vi "SMUVoltage.vi"() -> ()   [LabVIEW 2020]
uses:
  <instrlib>/niDCPower/nidcpower.llb/niDCPower Output Function.ctl
  <instrlib>/niDCPower/nidcpower.llb/niDCPower Measurement Type.ctl
panel:
  out "measurement":dbl format="%_6g"
  in  "instrument handle":refnum<k15>="NI_SMU1"
  in  "error in (no error)":errorcluster
  out "error out":errorcluster
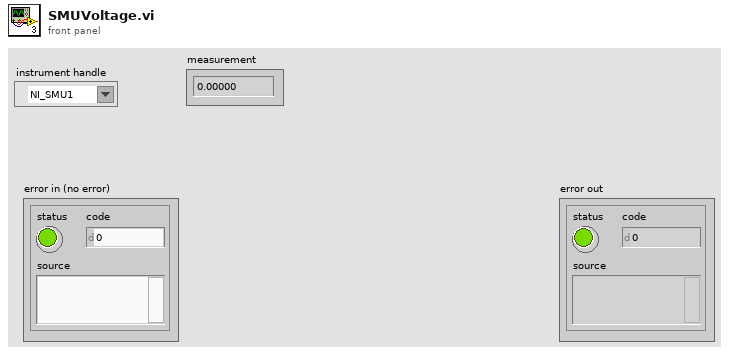
[diagram p1: front panel]
types:
  T1 = typedef "niDCPower Measurement Type.ctl" = i32
  T2 = typedef "niDCPower Output Function.ctl" = i32
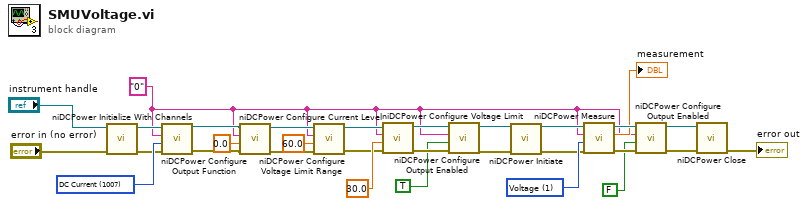
[diagram p0: block diagram]
diagram:
  w18 = T1 1 items=["Current", "Voltage"] ("measurement type")
  w2 = "0" ("channel name")
  w26 = T2 1007 items=["DC Voltage"=1006, "DC Current"=1007, "Pulse Voltage"=1049, "Pulse Current"=1050] ("output function")
  n1 = call <instrlib>:"niDCPower Initialize With Channels.vi"("error in (no error)"="error in (no error)", "resource name"="instrument handle") -> ("error out"=w25:errorcluster, "instrument handle out"=w27:refnum<k15>)  [unwired: 8 in]
  n2 = call <instrlib>:"niDCPower Configure Output Function.vi"("error in (no error)"=w25, "output function"=w26, "channel name"=w2, "instrument handle"=w27) -> ("error out"=w23:errorcluster, "instrument handle out"=w24:refnum<k15>)  [unwired: 6 in]
  n3 = call <instrlib>:"niDCPower Configure Current Level.vi"("error in (no error)"=w23, "current level"=0.0, "channel name"=w2, "instrument handle"=w24) -> ("error out"=w6:errorcluster, "instrument handle out"=w5:refnum<k15>)  [unwired: 6 in]
  n4 = call <instrlib>:"niDCPower Configure Voltage Limit Range.vi"("error in (no error)"=w6, "voltage limit range"=60.0, "channel name"=w2, "instrument handle"=w5) -> ("error out"=w3:errorcluster, "instrument handle out"=w4:refnum<k15>)  [unwired: 6 in]
  n5 = call <instrlib>:"niDCPower Configure Voltage Limit.vi"("error in (no error)"=w3, "voltage limit"=30.0, "channel name"=w2, "instrument handle"=w4) -> ("error out"=w21:errorcluster, "instrument handle out"=w20:refnum<k15>)  [unwired: 6 in]
  n6 = call <instrlib>:"niDCPower Configure Output Enabled.vi"("error in (no error)"=w21, "output enabled"=TRUE, "channel name"=w2, "instrument handle"=w20) -> ("error out"=w9:errorcluster, "instrument handle out"=w10:refnum<k15>)  [unwired: 6 in]
  n7 = call <instrlib>:"niDCPower Initiate.vi"("error in (no error)"=w9, "instrument handle"=w10) -> ("error out"=w8:errorcluster, "instrument handle out"=w7:refnum<k15>)  [unwired: 2 in, 6 out]
  n8 = call <instrlib>:"niDCPower Measure.vi"("error in (no error)"=w8, "measurement type"=w18, "channel name"=w2, "instrument handle"=w7) -> ("error out"=w17:errorcluster, "measurement"=→"measurement":dbl, "instrument handle out"=w16:refnum<k15>)  [unwired: 5 in]
  n9 = call <instrlib>:"niDCPower Configure Output Enabled.vi"("error in (no error)"=w17, "output enabled"=FALSE, "channel name"=w2, "instrument handle"=w16) -> ("error out"=w15:errorcluster, "instrument handle out"=w14:refnum<k15>)  [unwired: 6 in]
  n10 = call <instrlib>:"niDCPower Close.vi"("error in (no error)"=w15, "instrument handle"=w14) -> ("error out"=→"error out":errorcluster)  [unwired: 9 in]
